vi "PCO_Image_ColorSet.vi"() -> (0 "PCO_Image_ColorSet":T1, 1 "PCO_Image_ColorSet_Raw":T2, 2 "Length":u16, 3 "Raw_Length":u16)   [LabVIEW 2019, in "SDK.lvlib" / "Structures.lvlib"]
doc: "Use this template to build a VI to use as a subVI."
uses:
  Structures.lvlib
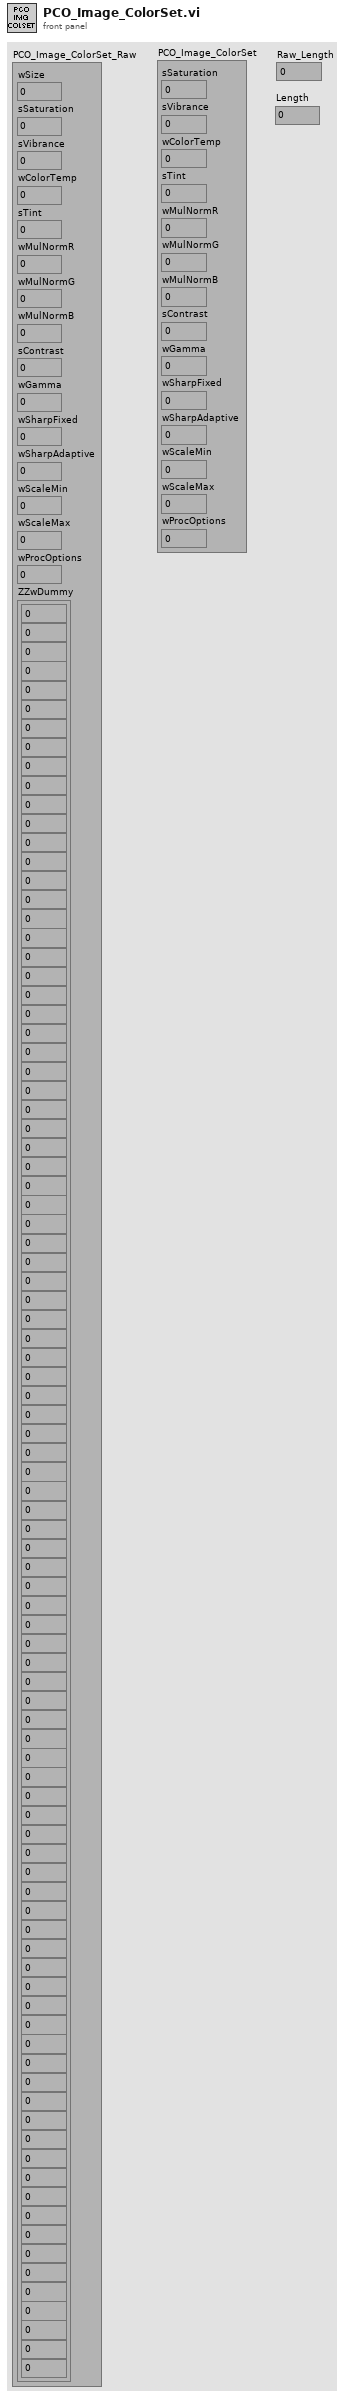
[diagram p1: front panel]
types:
  T1 = cluster{"sSaturation":i16, "sVibrance":i16, "wColorTemp":u16, "sTint":i16, "wMulNormR":u16, "wMulNormG":u16, "wMulNormB":u16, "sContrast":i16, "wGamma":u16, "wSharpFixed":u16, "wSharpAdaptive":u16, "wScaleMin":u16, "wScaleMax":u16, "wProcOptions":u16}
  T2 = cluster{"wSize":u16, "sSaturation":i16, "sVibrance":i16, "wColorTemp":u16, "sTint":i16, "wMulNormR":u16, "wMulNormG":u16, "wMulNormB":u16, "sContrast":i16, "wGamma":u16, "wSharpFixed":u16, "wSharpAdaptive":u16, "wScaleMin":u16, "wScaleMax":u16, "wProcOptions":u16, "ZZwDummy":cluster{u16, u16, u16, u16, u16, u16, u16, u16, u16, u16, u16, u16, u16, u16, u16, u16, u16, u16, u16, u16, u16, u16, u16, u16, u16, u16, u16, u16, u16, u16, u16, u16, u16, u16, u16, u16, u16, u16, u16, u16, u16, u16, u16, u16, u16, u16, u16, u16, u16, u16, u16, u16, u16, u16, u16, u16, u16, u16, u16, u16, u16, u16, u16, u16, u16, u16, u16, u16, u16, u16, u16, u16, u16, u16, u16, u16, u16, u16, u16, u16, u16, u16, u16, u16, u16, u16, u16, u16, u16, u16, u16, u16, u16}}
  T3 = cluster{u16, u16, u16, u16, u16, u16, u16, u16, u16, u16, u16, u16, u16, u16, u16, u16, u16, u16, u16, u16, u16, u16, u16, u16, u16, u16, u16, u16, u16, u16, u16, u16, u16, u16, u16, u16, u16, u16, u16, u16, u16, u16, u16, u16, u16, u16, u16, u16, u16, u16, u16, u16, u16, u16, u16, u16, u16, u16, u16, u16, u16, u16, u16, u16, u16, u16, u16, u16, u16, u16, u16, u16, u16, u16, u16, u16, u16, u16, u16, u16, u16, u16, u16, u16, u16, u16, u16, u16, u16, u16, u16, u16, u16}
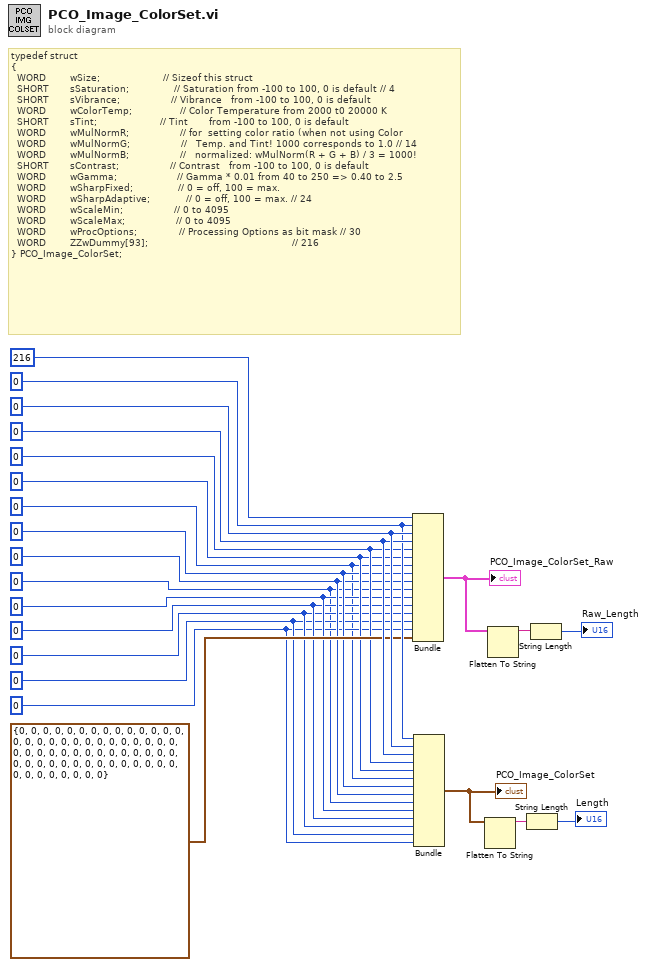
[diagram p0: block diagram]
diagram:
  w4 = u16 0 ("wProcOptions")
  w5 = u16 0 ("wScaleMax")
  w6 = u16 0 ("wScaleMin")
  w7 = u16 0 ("wSharpAdaptive")
  w8 = u16 0 ("wSharpFixed")
  w1 = u16 0 ("wGamma")
  w9 = i16 0 ("sContrast")
  w10 = u16 0 ("wMulNormB")
  w2 = u16 0 ("wMulNormG")
  w11 = u16 0 ("wMulNormR")
  w12 = i16 0 ("sTint")
  w15 = u16 0 ("wColorTemp")
  w16 = i16 0 ("sVibrance")
  w14 = i16 0 ("sSaturation")
  # "typedef struct\n{\n  WORD        wSize;                     // Sizeof this struct\n  SHORT       sSaturation;               // Saturation from -100 to 100, 0 is default // 4\n  SHORT       sVibrance;                 // Vibrance   from -100 to 100, 0 is default\n  WORD        wColorTemp;                // Color Temperature from 2000 t0 20000 K\n  SHORT       sTint;                     // Tint       from -100 to 100, 0 is default\n  WORD        wMulNormR;                 // for  setting color ratio (when not using Color\n  WORD        wMulNormG;                 //   Temp. and Tint! 1000 corresponds to 1.0 // 14\n  WORD        wMulNormB;                 //   normalized: wMulNorm(R + G + B) / 3 = 1000!\n  SHORT       sContrast;                 // Contrast   from -100 to 100, 0 is default\n  WORD        wGamma;                    // Gamma * 0.01 from 40 to 250 => 0.40 to 2.5\n  WORD        wSharpFixed;               // 0 = off, 100 = max.\n  WORD        wSharpAdaptive;            // 0 = off, 100 = max. // 24\n  WORD        wScaleMin;                 // 0 to 4095\n  WORD        wScaleMax;                 // 0 to 4095\n  WORD        wProcOptions;              // Processing Options as bit mask // 30\n  WORD        ZZwDummy[93];                                                // 216\n} PCO_Image_ColorSet;"
  n1 = Bundle("wSize"=u16 216, "sSaturation"=w14, "sVibrance"=w16, "wColorTemp"=w15, "sTint"=w12, "wMulNormR"=w11, "wMulNormG"=w2, "wMulNormB"=w10, "sContrast"=w9, "wGamma"=w1, "wSharpFixed"=w8, "wSharpAdaptive"=w7, "wScaleMin"=w6, "wScaleMax"=w5, "wProcOptions"=w4, "ZZwDummy"=T3 {0, 0, 0, 0, 0, 0, 0, 0, 0, 0, 0, 0, 0, 0, 0, 0, 0, 0, 0, 0, 0, 0, 0, 0, 0, 0, 0, 0, 0, 0, 0, 0, 0, 0, 0, 0, 0, 0, 0, 0, 0, 0, 0, 0, 0, 0, 0, 0, 0, 0, 0, 0, 0, 0, 0, 0, 0, 0, 0, 0, 0, 0, 0, 0, 0, 0, 0, 0, 0, 0, 0, 0, 0, 0, 0, 0, 0, 0, 0, 0, 0, 0, 0, 0, 0, 0, 0, 0, 0, 0, 0, 0, 0}) -> (w17:T2)  [unwired: 1 in]
  "PCO_Image_ColorSet_Raw" <- w17
  n2 = Bundle("sSaturation"=w14, "sVibrance"=w16, "wColorTemp"=w15, "sTint"=w12, "wMulNormR"=w11, "wMulNormG"=w2, "wMulNormB"=w10, "sContrast"=w9, "wGamma"=w1, "wSharpFixed"=w8, "wSharpAdaptive"=w7, "wScaleMin"=w6, "wScaleMax"=w5, "wProcOptions"=w4) -> (w3:T1)  [unwired: 1 in]
  "PCO_Image_ColorSet" <- w3
  n3 = Flatten To String(anything=w3) -> (data string=w22:string)  [unwired: 3 in, 2 out]
  n4 = Flatten To String(anything=w17) -> (data string=w21:string)  [unwired: 3 in, 2 out]
  n5 = String Length(string=w22) -> (length=→"Length":i32)
  n6 = String Length(string=w21) -> (length=→"Raw_Length":i32)
